vi "Robot Global Data.vi"() -> ()   [LabVIEW 2016]
doc: "This global VI can contain as many global variables as you need. Place a control on the panel, give it a good name. To read or write to it from a VI, drag the icon to the diagram of that VI. You can also drag from the project. Click on the node to change which global you access. You shouldn't have multiple locations writing to a global or it will cause a race-condition."
uses:
  <vilib>/Rock Robotics/WPI/Camera/WPI_CameraImageSize.ctl
  <vilib>/Rock Robotics/WPI/DriverStation/WPI_DriverStationRobotMode2.ctl
panel:
  in  "Right Encoder Distance":dbl
  in  "Left Encoder Distance":dbl
  in  "Gyro Angles":T1
  in  "Run Winch":bool
  in  "Winch Trigger":refnum<k4>
  in  "Hopper Dump Data":T2
  in  "Gear Dropper Data":T3
  in  "PID Right Motor Throttle":dbl
  in  "PID Left Motor Throttle":dbl
  in  "Right Encoder Rate":dbl(graph)
  in  "Left Encoder Rate":dbl(graph)
  in  "Gear Shift Data":T4
  in  "Simulated":bool
  in  "Robot Mode":T5
  in  "image size":T6=enum."320x240"
  in  "Enable Vision":bool
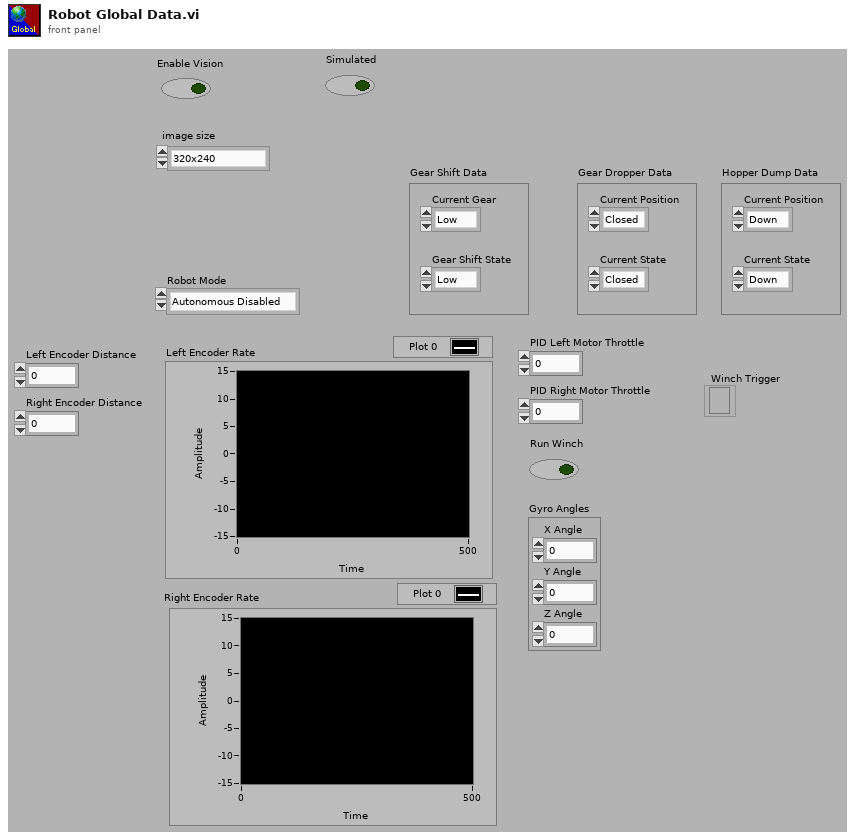
[diagram p1: front panel]
types:
  T1 = cluster{"X Angle":dbl, "Y Angle":dbl, "Z Angle":dbl}
  T2 = cluster{"Current Position":enum16{"Down", "Up"}, "Current State":enum16{"Down", "Shifting", "Up"}}
  T3 = cluster{"Current Position":enum16{"Closed", "Open"}, "Current State":enum16{"Closed", "Shifting", "Open"}}
  T4 = cluster{"Current Gear":enum16{"Low", "High"}, "Gear Shift State":enum16{"Low", "Shifting", "High"}}
  T5 = typedef "WPI_DriverStationRobotMode2.ctl" = enum16{"Autonomous Disabled", "Autonomous Enabled", "Teleop Disabled", "Teleop Enabled", "Disconnected", "Finish", "Test Disabled", "Test Enabled", "Emergency Stopped"}
  T6 = typedef "WPI_CameraImageSize.ctl" = enum16{"640x480", "320x240", "160x120", "Custom"}
diagram:
